vi "Untitled 1.vi"() -> ()   [LabVIEW 2024]
uses:
  <vilib>/measure/NI_MABase.lvlib
panel:
  out "Waveform Chart":waveform(dbl)(graph)
  in  "reset signal":bool
  in  "sampling info":cluster{"Fs":dbl, "#s":dbl}={"Fs"=1000.0, "#s"=1000.0} {"Fs" format="%.2p"}
  out "Y":dbl[](array[numeric])
  in  "stop":bool
  out "dt":dbl
  out "t0":timestamp
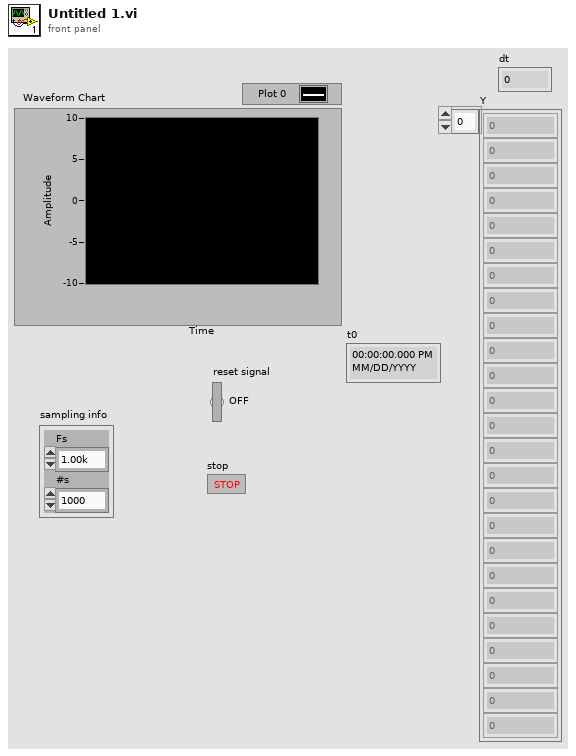
[diagram p1: front panel]
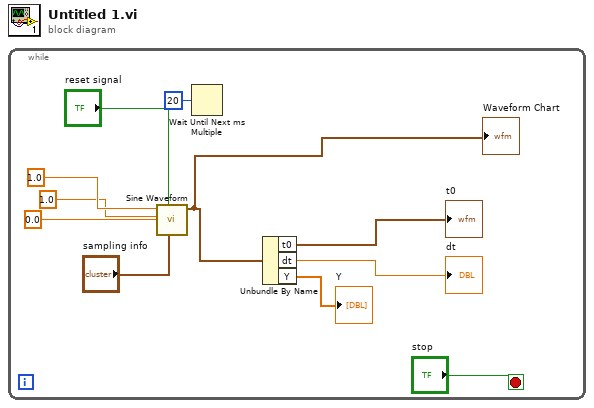
[diagram p0: block diagram]
diagram:
  n1 = while {
    stop <- "stop" stop-if-true
    n2 = call <vilib>:"Sine Waveform.vi"("offset"=0.0, "sampling info"="sampling info", "reset signal"="reset signal", "amplitude"=1.0, "frequency"=1.0) -> ("signal out"=w1:waveform(dbl))  [unwired: 5 in, 1 out]
    "Waveform Chart" <- w1
    n3 = Wait Until Next ms Multiple(millisecond multiple=u32 20) -> ()  [unwired: 1 out]
    n4 = Unbundle By Name(w1) -> ("t0"=→"t0":timestamp, "dt"=→"dt":dbl, "Y"=→"Y":dbl[])
  }
